vi "Builder.vi"() -> ()   [LabVIEW 2023]
uses:
  <vilib>/addons/_JKI Toolkits/State Machine/_JKI_lib_State_Machine.llb/Select State(s)_err__jki_lib_state_machine.vi
  <vilib>/AppBuilder/AB_API_Simple/Build (path).vi
  <userlib>/_OpenG.lib/appcontrol/appcontrol.llb/openg_application_control.lvlib
  <vilib>/AppBuilder/AB_API_Simple/NI_App_Builder_API.lvlib
panel:
  in  "BUILDER STATUS":i32(listbox)
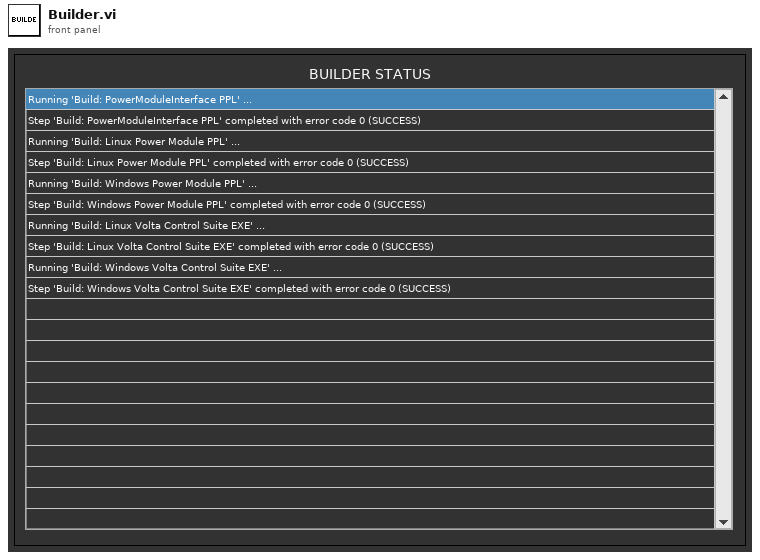
[diagram p1: front panel]
types:
  T1 = enum32{"Invalid", "Standard", "Closed", "Hidden", "Minimized", "Maximized"}
  T2 = enum32{"invalid app kind", "Development System", "Run Time System", "Student Edition", "Embedded LabVIEW", "Evaluation", "Custom"}
  T3 = cluster{"Core":cluster{"Current VI Reference":refnum<vi>, "Close Panel on Exit?":bool}}
  T4 = cluster{"Current VI Reference":refnum<vi>, "Close Panel on Exit?":bool}
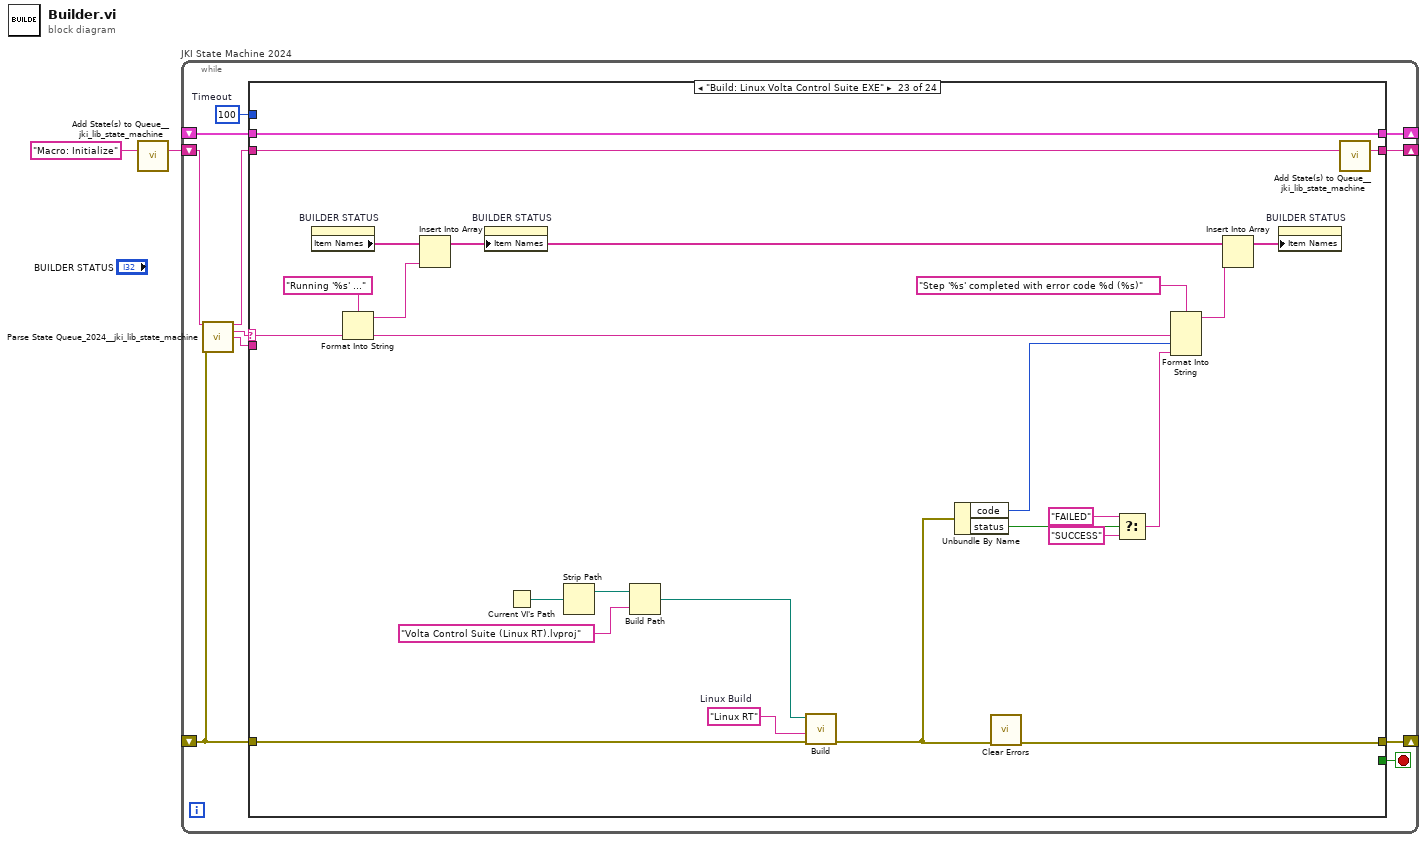
[diagram p0: block diagram]
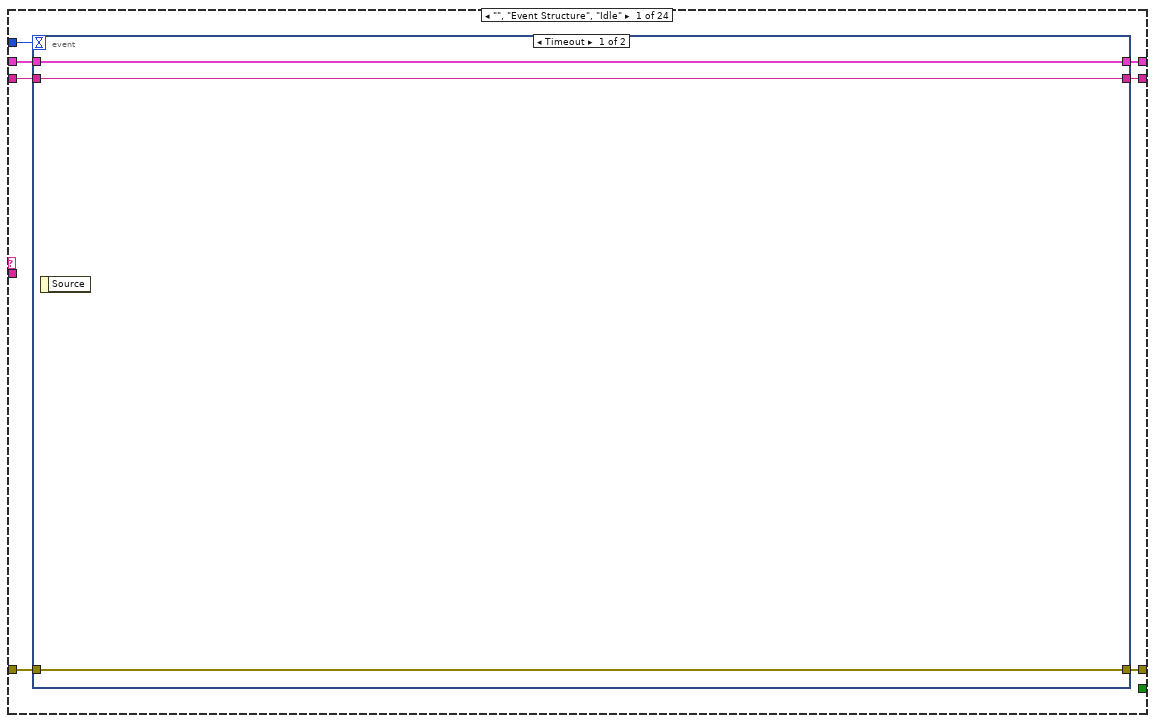
[diagram p2: hidden frame]
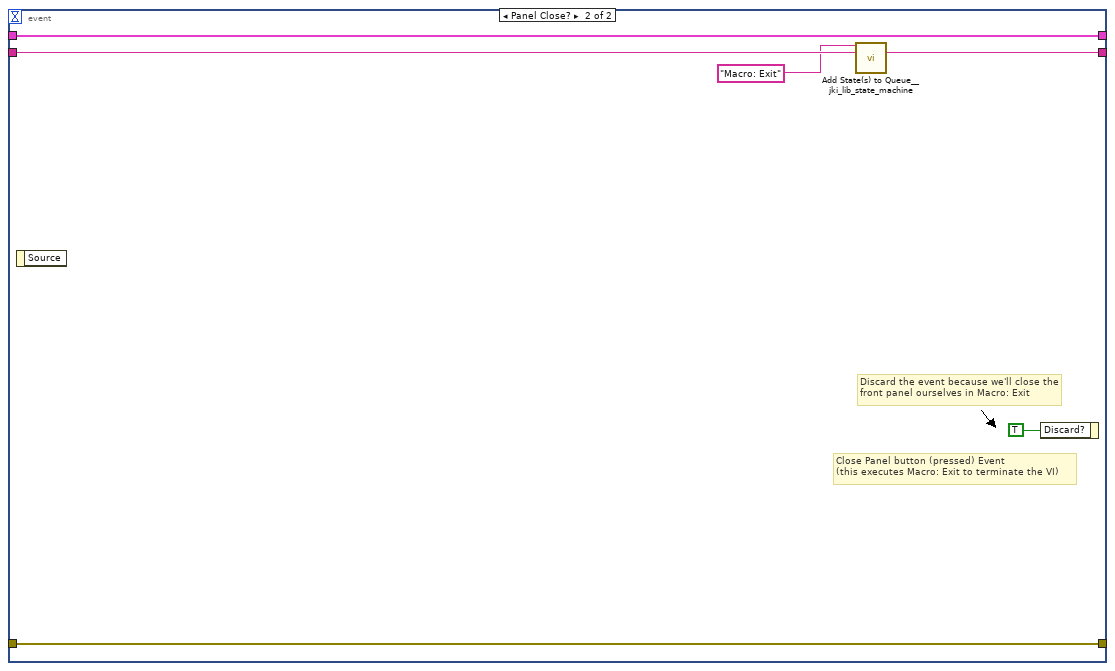
[diagram p3: hidden frame]
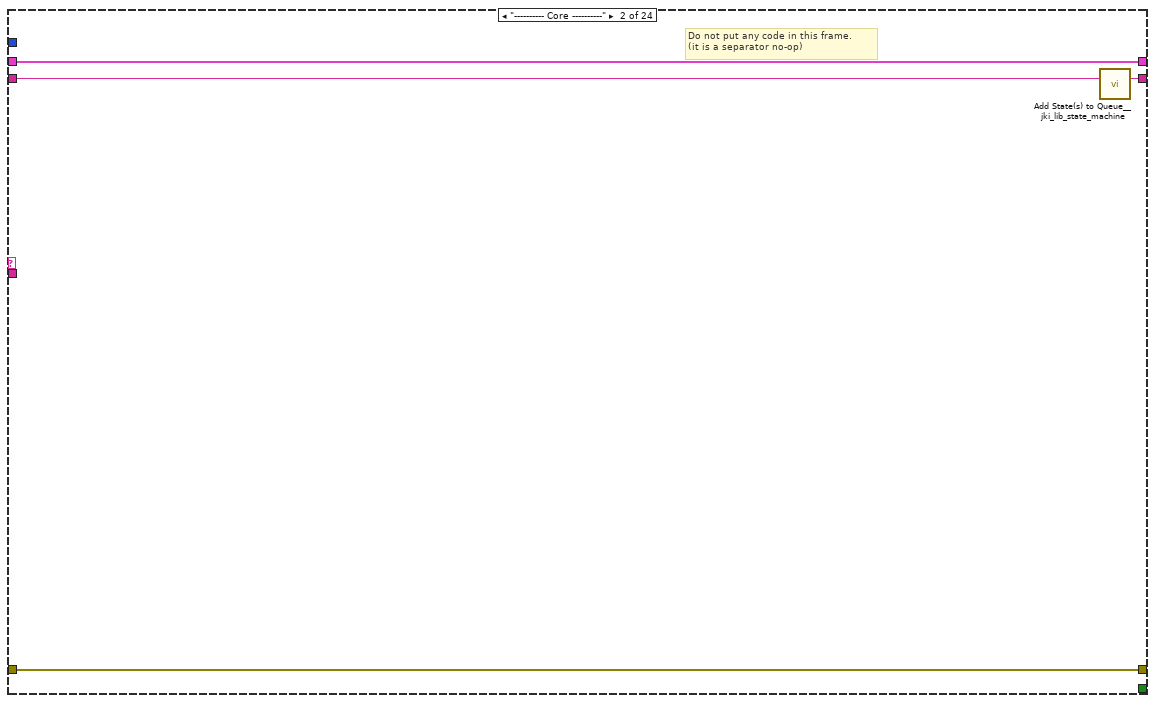
[diagram p4: hidden frame]
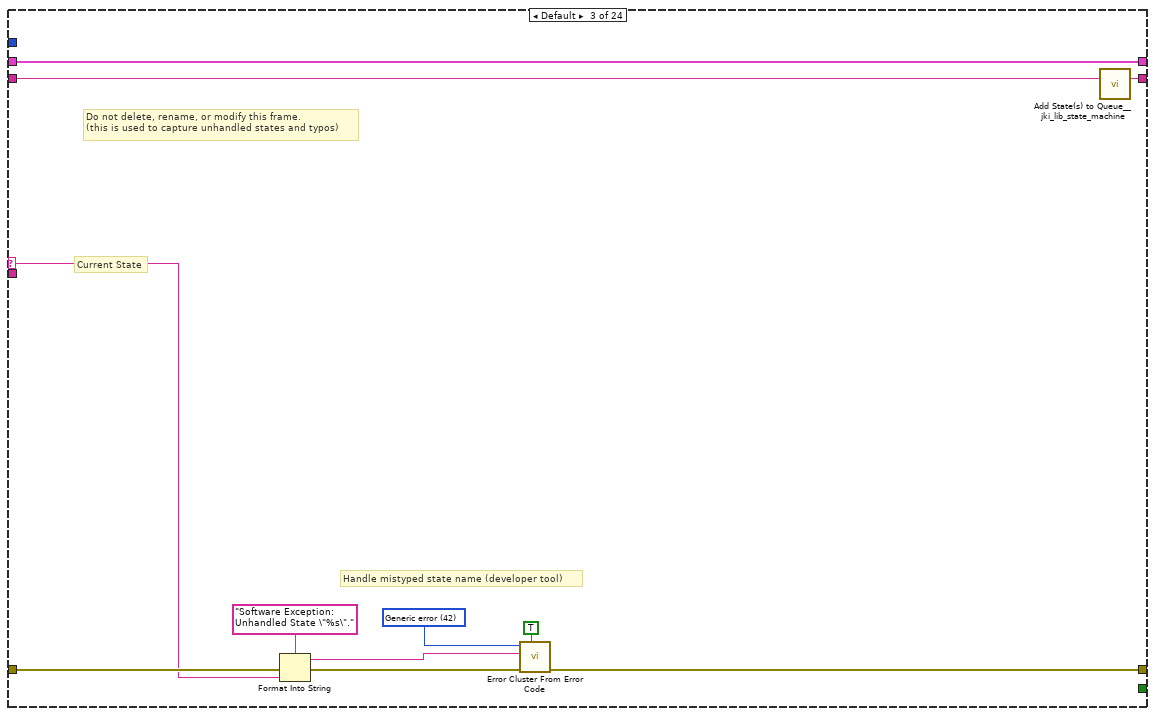
[diagram p5: hidden frame]
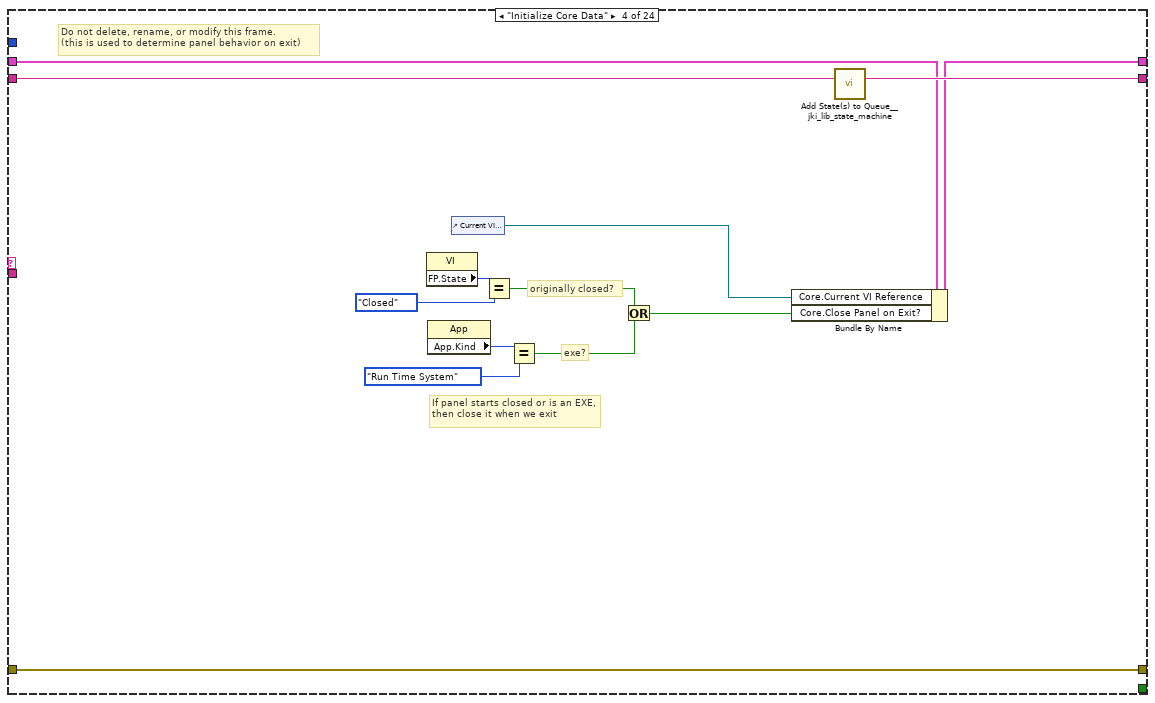
[diagram p6: hidden frame]
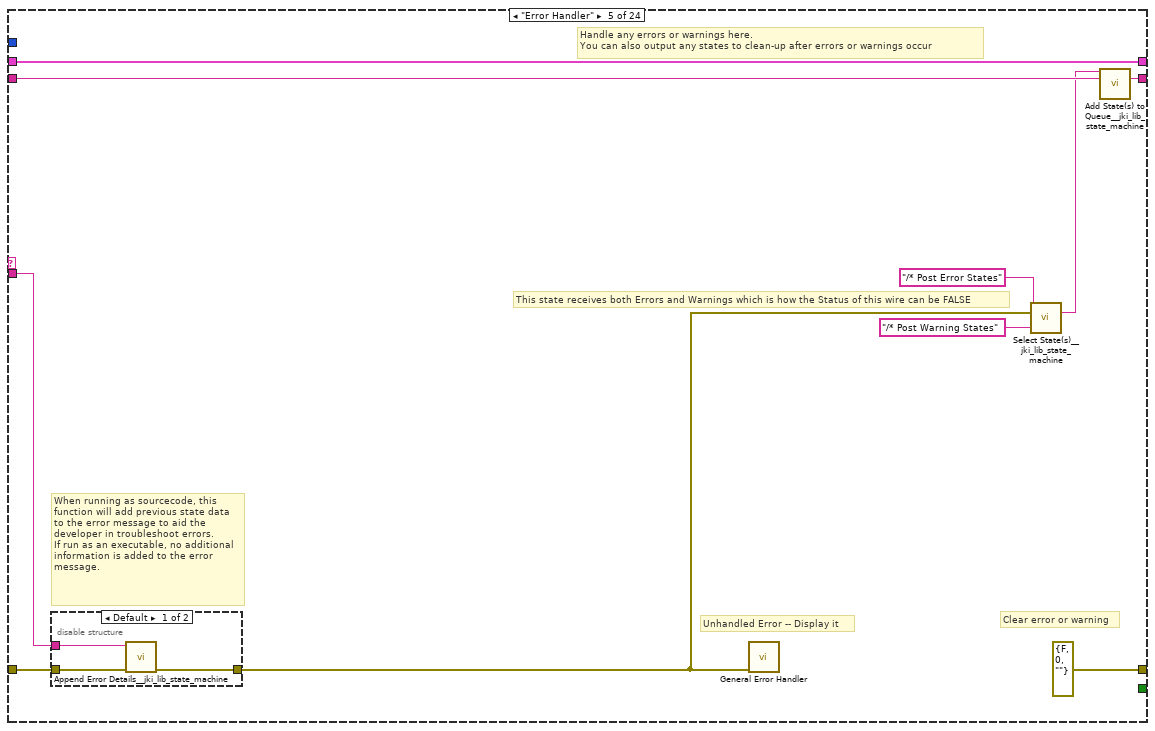
[diagram p7: hidden frame]
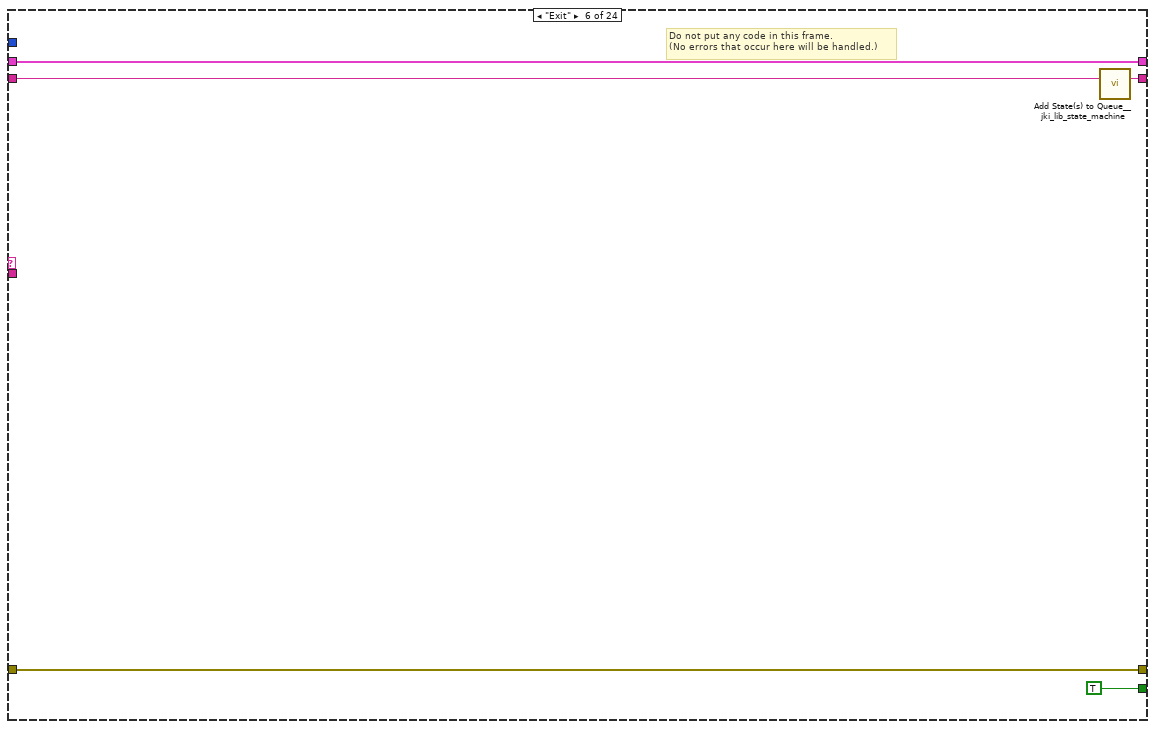
[diagram p9: hidden frame]
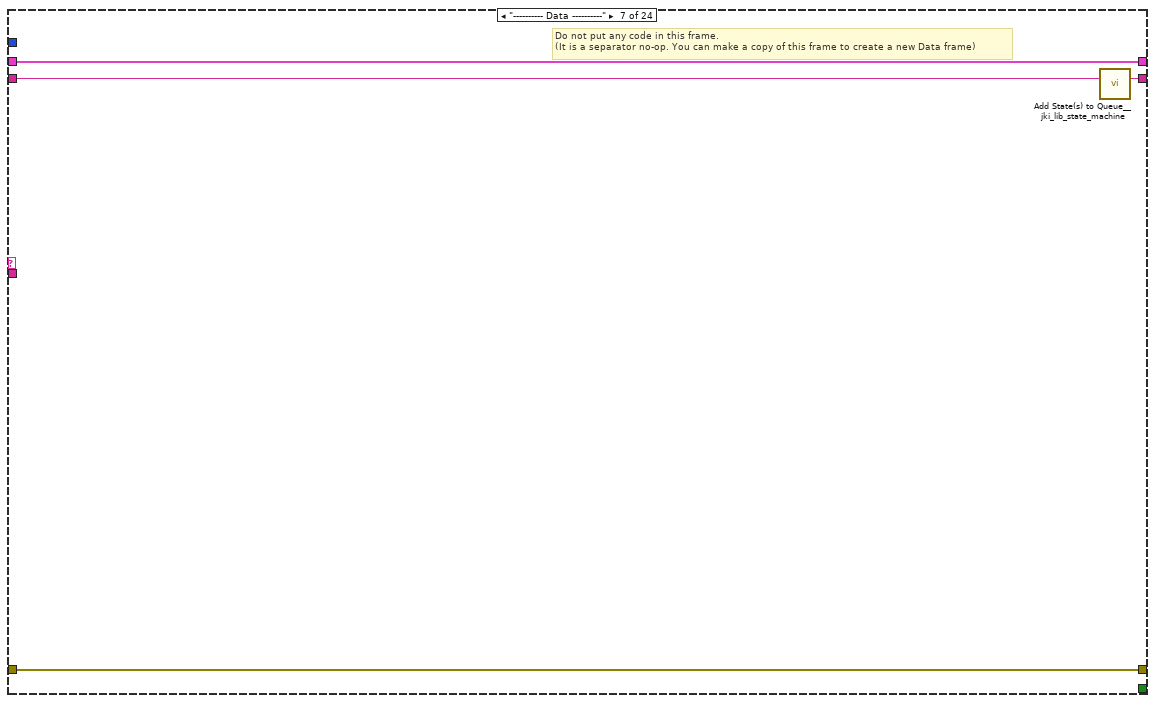
[diagram p10: hidden frame]
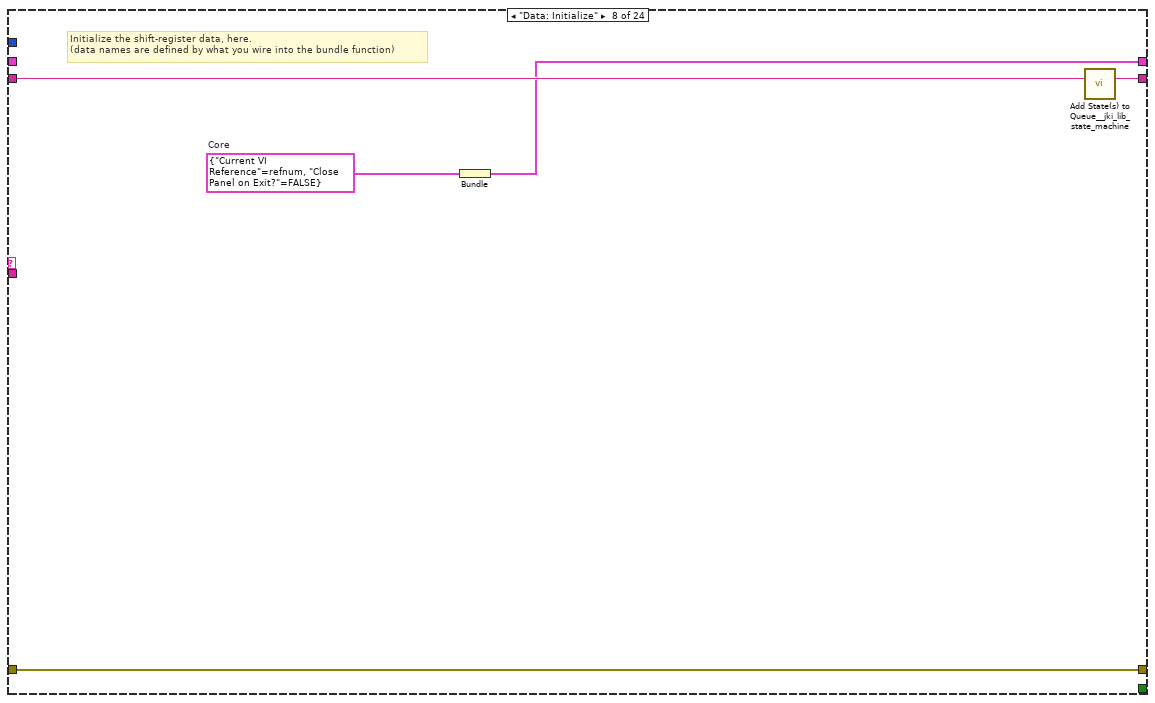
[diagram p11: hidden frame]
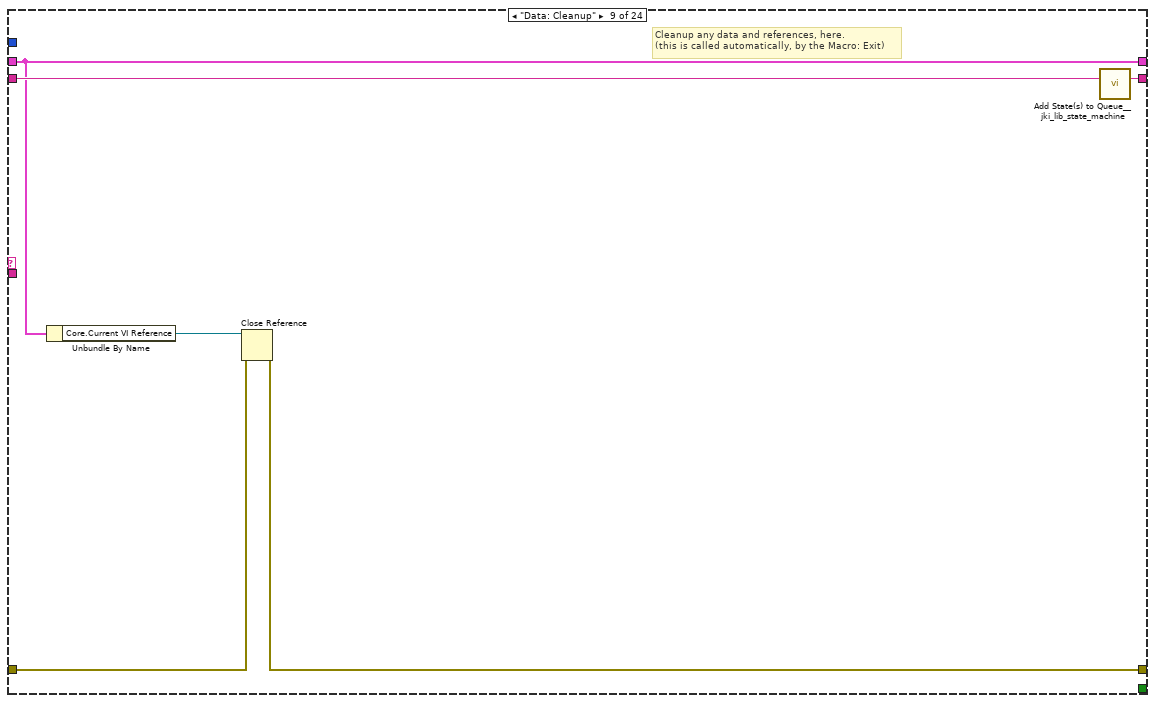
[diagram p12: hidden frame]
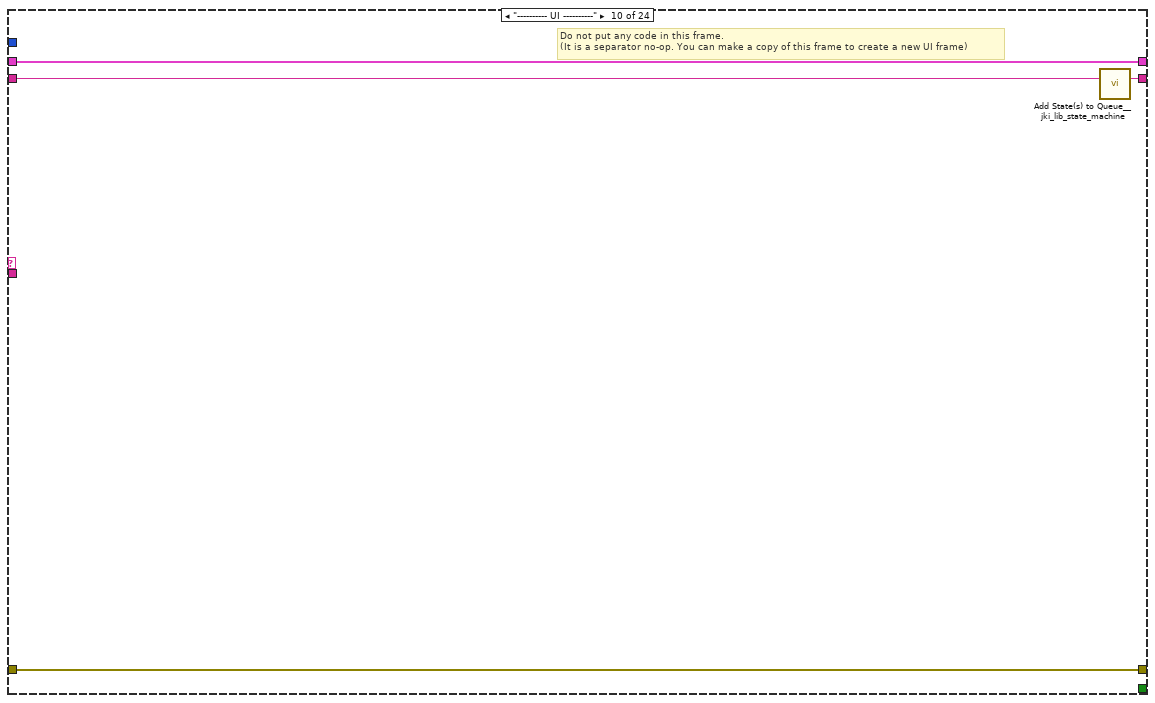
[diagram p13: hidden frame]
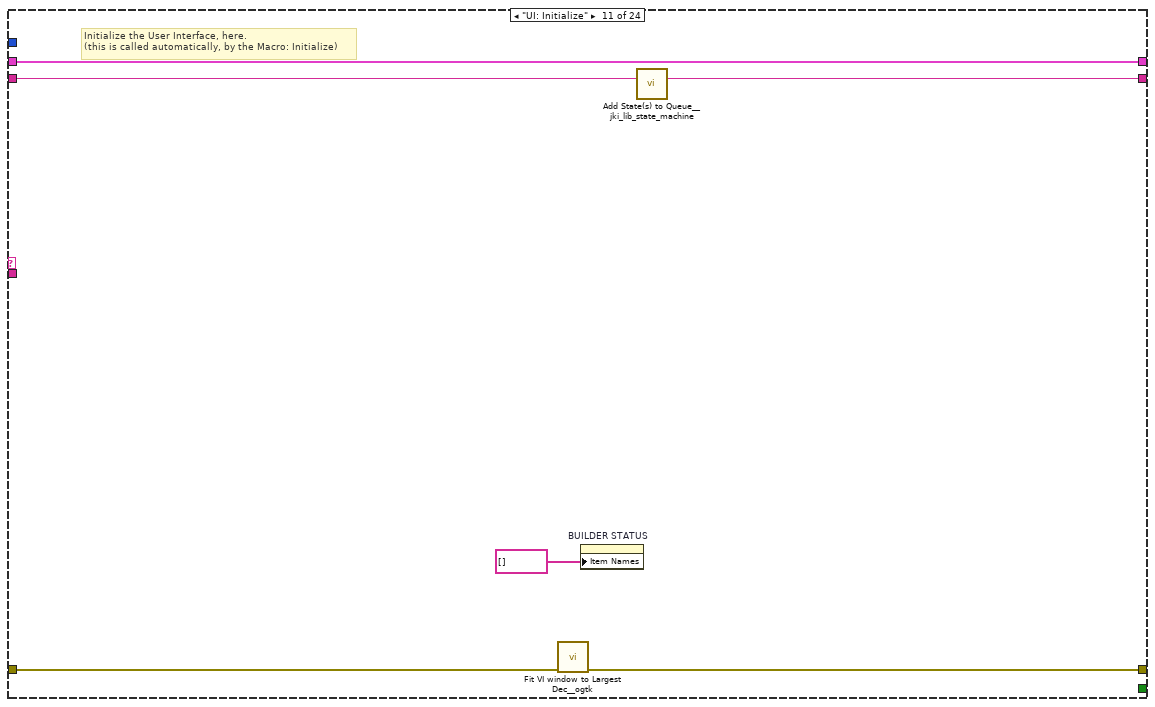
[diagram p14: hidden frame]
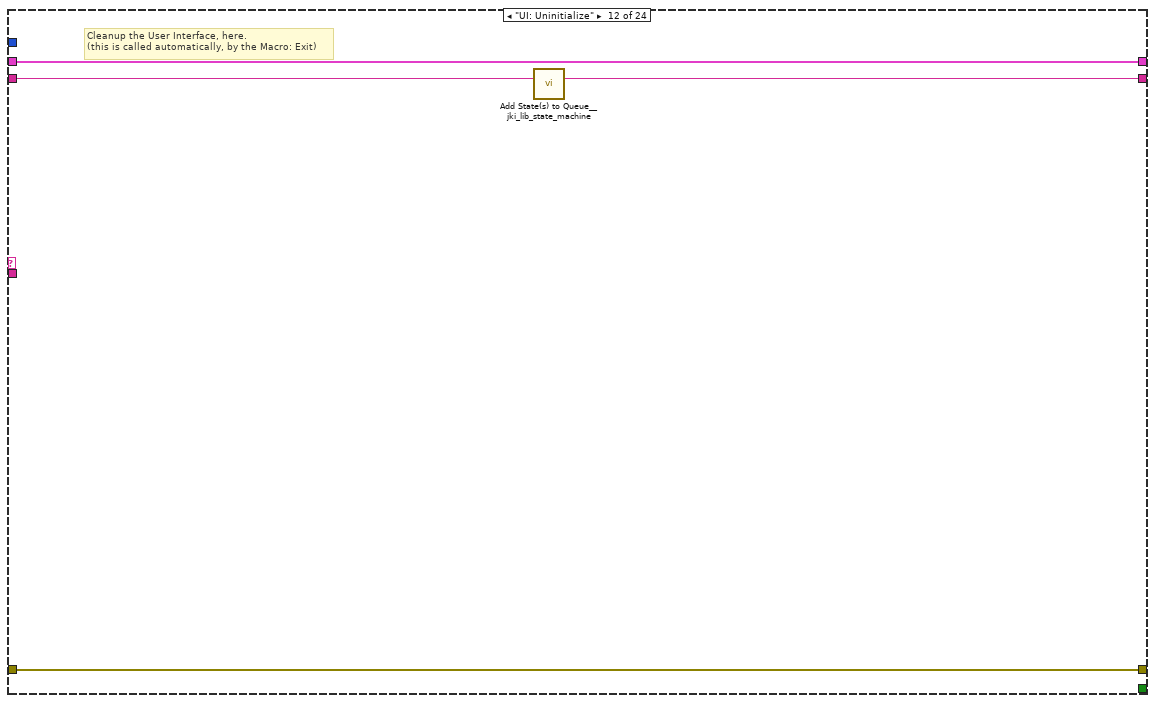
[diagram p15: hidden frame]
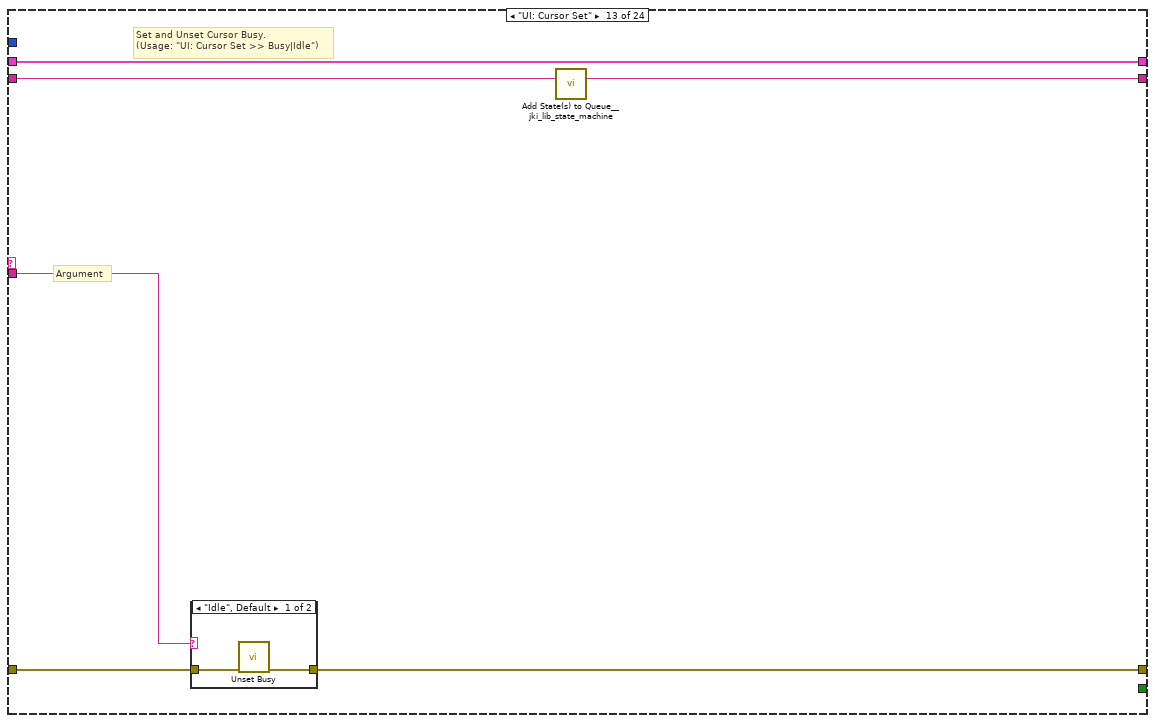
[diagram p16: hidden frame]
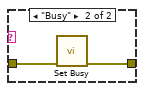
[diagram p17: hidden frame]
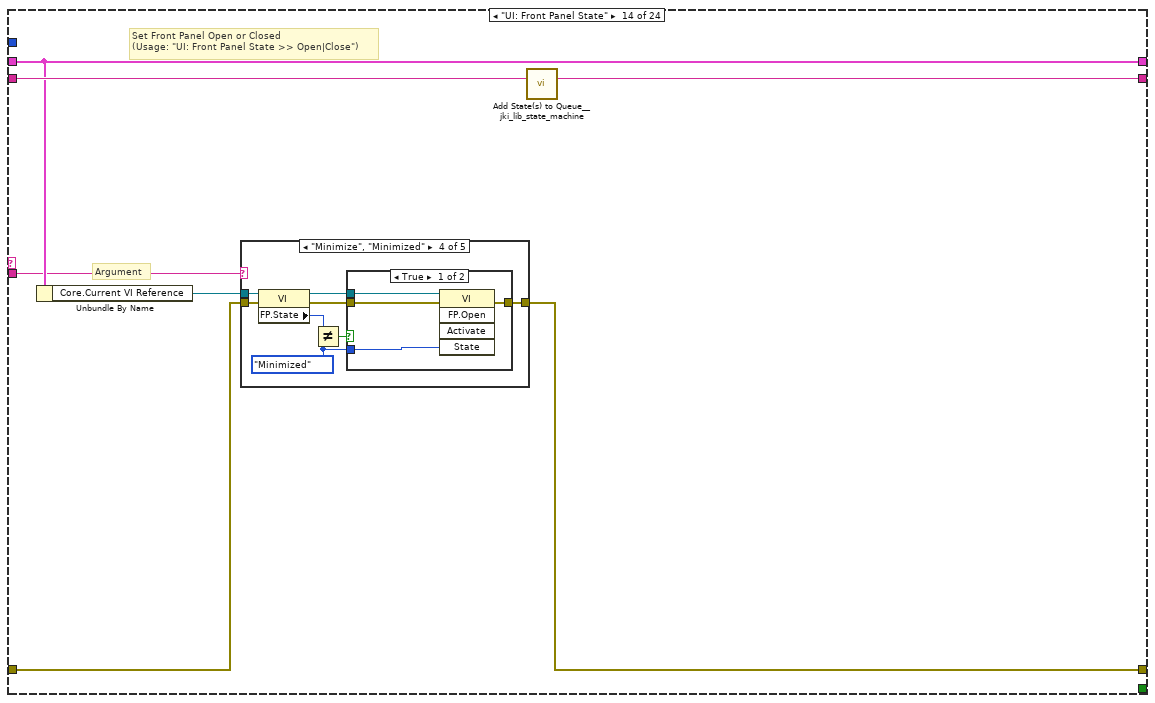
[diagram p18: hidden frame]
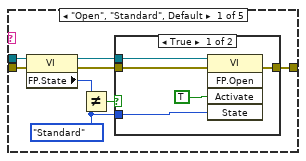
[diagram p19: hidden frame]
diagram:
  n1 = call <vilib>:"Add State(s) to Queue__jki_lib_state_machine.vi"("State(s) in (\"\")"="Macro: Initialize") -> ("States Out"=w2:string)  [unwired: 14 in]
  n2 = while "JKI State Machine 2024" {
    shift-right: [w6] -> _
    shift-left: _ -> [w5]
    shift-right: [w9] -> _
    shift-left: _ -> [w3]
    shift-right: [w8] -> _
    shift-left: w2 -> [w10]
    stop <- w7 stop-if-true
    w4 = 100  # Timeout
    n3 = call <vilib>:"Parse State Queue_2024__jki_lib_state_machine.vi"("State Queue"=w10, "Error In (no error)"=w3) -> ("Remaining States"=w12:string, "Current State"=w13:string, "Arguments"=w11:string)  [unwired: 11 in]
    n4 = case shown="\"Build: Linux Volta Control Suite EXE\"" w13 {
      selector: w13 -> [_ _ w34 _ _ _ _ _ _ _ _ _ _ _ _ _ _ _ _ w230 w253 w277 w301 w325]
      tunnel: w12 -> [w20 w33 w38 w57 w67 w76 w80 w85 w91 w95 w101 w105 w111 w122 w191 w196 w201 w206 w210 w238 w262 w286 w310 w334]
      tunnel: w11 -> [_ _ _ _ w62 _ _ _ _ _ _ _ w106 w116 _ _ _ _ _ _ _ _ _ _]
      tunnel: w5 -> [w18 w30 w36 w50 w64 w74 w77 _ w86 w92 w99 w103 w109 w118 w188 w193 w198 w204 w207 w236 w260 w284 w308 w332]
      tunnel: [w17 w31 w40 w54 errorcluster {"status"=FALSE, "code"=0, "source"=""} ("error out") w73 w78 w82 w87 w93 w96 w102 w107 w119 w189 w194 w199 w203 w208 w218 w246 w270 w294 w318] -> w9
      tunnel: w3 -> [w14 w31 w39 w54 w63 w73 w78 w82 w88 w93 w98 w102 w108 w120 w189 w194 w199 w203 w208 w225 w244 w268 w292 w316]
      tunnel: [w19 w32 w37 w56 w66 w75 w79 w84 w90 w94 w100 w104 w110 w121 w190 w195 w200 w205 w209 w237 w261 w285 w309 w333] -> w8
      tunnel: [_ _ _ _ _ TRUE _ _ _ _ _ _ _ _ _ _ _ _ _ _ _ _ _ _] -> w7
      tunnel: [w16 w30 w36 w55 w64 w74 w77 w83 w86 w92 w99 w103 w109 w118 w188 w193 w198 w204 w207 w236 w260 w284 w308 w332] -> w6
      tunnel: w4 -> [w15 _ _ _ _ _ _ _ _ _ _ _ _ _ _ _ _ _ _ _ _ _ _ _]
      frame "", "Event Structure", "Idle" {
        n5 = event shown="[0] Timeout" {
          selector: _ -> [_ _]
          dyn-events: _ -> [_ _]
          timeout: w15 -> [_ _]
          tunnel: w20 -> [w21 w29]
          tunnel: [w21 w28] -> w19
          tunnel: w18 -> [w22 w26]
          tunnel: [w23 w27] -> w17
          tunnel: w14 -> [w23 w27]
          tunnel: [w22 w26] -> w16
          event Timeout {
            n6 = event-data() -> ()  [unwired: 1 in, 1 out]
          }
          event Panel Close? {
            # "Discard the event because we'll close the front panel ourselves in Macro: Exit"
            # "Close Panel button (pressed) Event\n(this executes Macro: Exit to terminate the VI)"
            n7 = event-data() -> ()  [unwired: 1 in, 1 out]
            n8 = call <vilib>:"Add State(s) to Queue__jki_lib_state_machine.vi"("State(s) in Front (\"\")"="Macro: Exit", "State(s) in (\"\")"=w29) -> ("States Out"=w28:string)  [unwired: 13 in]
            n9 = event-data("Discard?"=TRUE) -> ()  [unwired: 1 in, 1 out]
          }
        }
      }
      frame "---------- Core ----------" {
        # "Do not put any code in this frame.\n(it is a separator no-op)"
        n10 = call <vilib>:"Add State(s) to Queue__jki_lib_state_machine.vi"("State(s) in (\"\")"=w33) -> ("States Out"=w32:string)  [unwired: 14 in]
      }
      frame Default {
        w43 = 42 items=["No error", "Argument error", "Memory is full", "Out of zone", "End of file", "File already open", "Generic file I/O error", "File not found", "File permission error", "Disk is full", "Duplicate path", "Too many files open", "System feature not enabled", "Resource file not found", "Cannot add resource", "Resource not found", "Image not found", "Image memory error", "Pen does not exist", "Config type invalid", "Config token not found", "Config parse error", "Config memory error", "Bad external code format", "Bad external code offset", "External code not present", "Null window", "Destroy window error", "Null menu", "Print aborted", "Bad print record", "Print driver error", "Windows error during printing", "Memory error during printing", "Print dialog error", "Generic print error", "Invalid device refnum", "Device not found", "Device parameter error", "Device unit error", "Cannot open device", "Device call aborted", "Generic error", "Cancelled by user", "Object ID too low", "Object ID too high", "Object not in heap", "Unknown heap", "Unknown object (invalid DefProc)", "Unknown object (DefProc not in table)", "Message out of range", "Invalid (null) method", "Unknown message", "Manager call not supported", "Bad address", "Network operation in progress", "Network operation timed out", "Connection is busy", "Network attribute not supported", "Network error", "Address in use", "System out of memory", "Connection aborted", "Connection refused", "Not connected", "Already connected", "Connection closed", "Initialization error (interapplication manager)", "Bad occurrence", "Wait on unbound occurrence handler", "Occurrence queue overflow", "Datalog type conflict", "Unused", "Unrecognized type (interapplication manager)", "Memory corrupt", "Failed to make temporary DLL", "Old CIN version", "Drag socket not found", "Failed to load drop-object", "Failed to register OLE object", "Failed to release OLE object", "Format specifier type mismatch", "Unknown format specifier", "Too few format specifiers", "Too many format specifiers", "Scan failed", "Newer CIN version", "Error converting to variant", "Runtime menu error", "Password tampered", "Variant attribute not found", "Incompatible variant data type", "Event data is not available", "Event Store is not present", "Occurrence is not found", "Event Queue is not created", "Event info is not available", "Refnum passed is NULL", "Error retrieving Class GUID", "Error retrieving CoClass GUID", "Error retrieving TypeLib GUID.", "Bad built application magic bytes.", "Specific driver is different from the specific driver associated with the Logical Name.", "There is no session opened to the class driver.", "Max Error", "MAX - Error with config objects", "MAX - Error loading configuration", "MAX - Group not supported"]
        # "Current State"
        # "Do not delete, rename, or modify this frame.\n(this is used to capture unhandled states and typos)"
        # "Handle mistyped state name (developer tool)"
        n11 = Format Into String(format string="Software Exception: Unhandled State \"%s\"." ("message"), error in=w39, w34) -> (resulting string=w42:string, error out=w41:errorcluster)  [unwired: 1 in]
        n12 = call <vilib>:"Error Cluster From Error Code.vi"("show call chain? (False)"=TRUE, "error in (no error)"=w41, "error message (\"\")"=w42, "error code (0)"=w43) -> ("error out"=w40:errorcluster)  [unwired: 5 in]
        n13 = call <vilib>:"Add State(s) to Queue__jki_lib_state_machine.vi"("State(s) in (\"\")"=w38) -> ("States Out"=w37:string)  [unwired: 14 in]
      }
      frame "Initialize Core Data" {
        # "Do not delete, rename, or modify this frame.\n(this is used to determine panel behavior on exit)"
        # "originally closed?"
        # "exe?"
        # "If panel starts closed or is an EXE, then close it when we exit"
        n14 = property class="VI"() -> ("FP.State"=w47:T1)  [unwired: 2 in, 2 out]
        n15 = property class="App"() -> ("App.Kind"=w53:T2)  [unwired: 2 in, 2 out]
        n16 = control-ref of="Current VI Reference"() -> (w48:refnum<vi>)
        n17 = Equal?(x=w47, y=T1."Closed" ("Front Panel Window:State")) -> (x = y?=w45:bool)
        n18 = Equal?(x=w53, y=T2."Run Time System" ("Application:Kind")) -> (x = y?=w51:bool)
        n19 = Or(x=w45, y=w51) -> (x .or. y?=w49:bool)
        n20 = Bundle By Name(cluster=w50, "Core.Current VI Reference"=w48, "Core.Close Panel on Exit?"=w49) -> (w55:T3)
        n21 = call <vilib>:"Add State(s) to Queue__jki_lib_state_machine.vi"("State(s) in (\"\")"=w57) -> ("States Out"=w56:string)  [unwired: 14 in]
      }
      frame "Error Handler" {
        # "When running as sourcecode, this function will add previous state data to the error message to aid the developer in troubleshoot errors.\nIf run as an executable, no additional information is added to the error message."
        # "This state receives both Errors and Warnings which is how the Status of this wire can be FALSE"
        # "Unhandled Error -- Display it"
        # "Handle any errors or warnings here.\nYou can also output any states to clean-up after errors or warnings occur"
        # "Clear error or warning"
        n22 = disable-structure shown="Default" {
          disable-tunnel: w63 -> [w70 w71]
          disable-tunnel: w62 -> [w69 _]
          disable-tunnel: [w68 w71] -> w61
          frame condition #0 (active) {
            n23 = call <vilib>:"Append Error Details__jki_lib_state_machine.vi"("error in (no error)"=w70, "Previous State and Argument(s)"=w69) -> ("error out"=w68:errorcluster)  [unwired: 9 in]
          }
          frame condition #1 {
          }
        }
        n24 = call <vilib>:"General Error Handler.vi"("error in (no error)"=w61) -> ()  [unwired: 10 in, 5 out]
        n25 = call-poly <vilib>:"Select State(s)__jki_lib_state_machine.vi"("State(s) if True (\"\")"="/* Post Error States", "Select"=w61, "State(s) if False (\"\")"="/* Post Warning States") -> ("States Out"=w59:string)  [unwired: 12 in]
        n26 = call <vilib>:"Add State(s) to Queue__jki_lib_state_machine.vi"("State(s) in Front (\"\")"=w59, "State(s) in (\"\")"=w67) -> ("States Out"=w66:string)  [unwired: 13 in]
      }
      frame "Exit" {
        # "Do not put any code in this frame.\n(No errors that occur here will be handled.)"
        n27 = call <vilib>:"Add State(s) to Queue__jki_lib_state_machine.vi"("State(s) in (\"\")"=w76) -> ("States Out"=w75:string)  [unwired: 14 in]
      }
      frame "---------- Data ----------" {
        # "Do not put any code in this frame.\n(It is a separator no-op. You can make a copy of this frame to create a new Data frame)"
        n28 = call <vilib>:"Add State(s) to Queue__jki_lib_state_machine.vi"("State(s) in (\"\")"=w80) -> ("States Out"=w79:string)  [unwired: 14 in]
      }
      frame "Data: Initialize" {
        w81 = T4 {"Current VI Reference"=refnum, "Close Panel on Exit?"=FALSE}  # Core
        # "Initialize the shift-register data, here.\n(data names are defined by what you wire into the bundle function)"
        n29 = Bundle("Core"=w81) -> (w83:T3)  [unwired: 1 in]
        n30 = call <vilib>:"Add State(s) to Queue__jki_lib_state_machine.vi"("State(s) in (\"\")"=w85) -> ("States Out"=w84:string)  [unwired: 14 in]
      }
      frame "Data: Cleanup" {
        # "Cleanup any data and references, here.\n(this is called automatically, by the Macro: Exit)"
        n31 = Unbundle By Name(w86) -> ("Core.Current VI Reference"=w89:refnum<vi>)
        n32 = Close Reference(reference=w89, error in (no error)=w88) -> (error out=w87:errorcluster)
        n33 = call <vilib>:"Add State(s) to Queue__jki_lib_state_machine.vi"("State(s) in (\"\")"=w91) -> ("States Out"=w90:string)  [unwired: 14 in]
      }
      frame "---------- UI ----------" {
        # "Do not put any code in this frame.\n(It is a separator no-op. You can make a copy of this frame to create a new UI frame)"
        n34 = call <vilib>:"Add State(s) to Queue__jki_lib_state_machine.vi"("State(s) in (\"\")"=w95) -> ("States Out"=w94:string)  [unwired: 14 in]
      }
      frame "UI: Initialize" {
        # "Initialize the User Interface, here.\n(this is called automatically, by the Macro: Initialize)"
        n35 = call <userlib>:"Fit VI window to Largest Dec__ogtk.vi"("error in (no error)"=w98) -> ("error out"=w96:errorcluster)  [unwired: 5 in, 1 out]
        n36 = property on="BUILDER STATUS" class="LstBox (strict)"("Item Names"=string[] []) -> ()  [unwired: 2 in, 2 out]
        n37 = call <vilib>:"Add State(s) to Queue__jki_lib_state_machine.vi"("State(s) in (\"\")"=w101) -> ("States Out"=w100:string)  [unwired: 14 in]
      }
      frame "UI: Uninitialize" {
        # "Cleanup the User Interface, here.\n(this is called automatically, by the Macro: Exit)"
        n38 = call <vilib>:"Add State(s) to Queue__jki_lib_state_machine.vi"("State(s) in (\"\")"=w105) -> ("States Out"=w104:string)  [unwired: 14 in]
      }
      frame "UI: Cursor Set" {
        # "Argument"
        # "Set and Unset Cursor Busy.\n(Usage: \"UI: Cursor Set >> Busy|Idle\")"
        n39 = case shown="\"Idle\", Default" w106 {
          tunnel: w108 -> [w113 w115]
          tunnel: [w112 w114] -> w107
          frame "Idle", Default {
            n40 = call <vilib>:"Unset Busy.vi"("error in (no error)"=w113) -> ("error out"=w112:errorcluster)  [unwired: 10 in]
          }
          frame "Busy" {
            n41 = call <vilib>:"Set Busy.vi"("error in (no error)"=w115) -> ("error out"=w114:errorcluster)  [unwired: 9 in, 1 out]
          }
        }
        n42 = call <vilib>:"Add State(s) to Queue__jki_lib_state_machine.vi"("State(s) in (\"\")"=w111) -> ("States Out"=w110:string)  [unwired: 14 in]
      }
      frame "UI: Front Panel State" {
        # "Argument"
        # "Set Front Panel Open or Closed\n(Usage: \"UI: Front Panel State >> Open|Close\")"
        n43 = Unbundle By Name(w118) -> ("Core.Current VI Reference"=w117:refnum<vi>)
        n44 = case shown="\"Minimize\", \"Minimized\"" w116 {
          tunnel: w120 -> [w128 w143 w154 w167 w180]
          tunnel: [w130 w144 w156 w169 w182] -> w119
          tunnel: w117 -> [w129 w141 w155 w168 w181]
          frame "Open", "Standard", Default {
            w123 = T1."Standard" ("State")
            n45 = property class="VI"(reference=w129, error in=w128) -> (reference out=w126:refnum<vi>, error out=w127:errorcluster, "FP.State"=w125:T1)
            n46 = Not Equal?(x=w125, y=w123) -> (x != y?=w124:bool)
            n47 = case shown="True" w124 {
              tunnel: [w134 w136] -> w130
              tunnel: w127 -> [w133 w136]
              tunnel: w126 -> [w132 _]
              tunnel: w123 -> [w131 _]
              frame True {
                n48 = invoke class="VI" method="FP.Open"(reference=w132, error in=w133, "Activate"=TRUE, "State"=w131) -> (error out=w134:errorcluster)  [unwired: 1 in, 4 out]
              }
              frame False {
              }
            }
          }
          frame "Close", "Closed" {
            n49 = property class="VI"(reference=w141, error in=w143) -> (reference out=w140:refnum<vi>, error out=w142:errorcluster, "FP.State"=w138:T1)
            n50 = Not Equal?(x=w138, y=T1."Closed" ("Front Panel Window:State")) -> (x != y?=w137:bool)
            n51 = case shown="True" w137 {
              tunnel: [w145 w148] -> w144
              tunnel: w142 -> [w145 w147]
              tunnel: w140 -> [_ w146]
              frame False {
              }
              frame True {
                n52 = invoke class="VI" method="FP.Close"(reference=w146, error in=w147) -> (error out=w148:errorcluster)  [unwired: 1 in, 2 out]
              }
            }
          }
          frame "Hidden", "Hide" {
            w149 = T1."Hidden" ("State")
            n53 = property class="VI"(reference=w155, error in=w154) -> (reference out=w152:refnum<vi>, error out=w153:errorcluster, "FP.State"=w151:T1)
            n54 = Not Equal?(x=w151, y=w149) -> (x != y?=w150:bool)
            n55 = case shown="True" w150 {
              tunnel: [w160 w161] -> w156
              tunnel: w153 -> [w159 w161]
              tunnel: w152 -> [w158 _]
              tunnel: w149 -> [w157 _]
              frame True {
                n56 = invoke class="VI" method="FP.Open"(reference=w158, error in=w159, "State"=w157) -> (error out=w160:errorcluster)  [unwired: 2 in, 4 out]
              }
              frame False {
              }
            }
          }
          frame "Minimize", "Minimized" {
            w162 = T1."Minimized" ("State")
            n57 = property class="VI"(reference=w168, error in=w167) -> (reference out=w165:refnum<vi>, error out=w166:errorcluster, "FP.State"=w164:T1)
            n58 = Not Equal?(x=w164, y=w162) -> (x != y?=w163:bool)
            n59 = case shown="True" w163 {
              tunnel: [w173 w174] -> w169
              tunnel: w166 -> [w172 w174]
              tunnel: w165 -> [w171 _]
              tunnel: w162 -> [w170 _]
              frame True {
                n60 = invoke class="VI" method="FP.Open"(reference=w171, error in=w172, "State"=w170) -> (error out=w173:errorcluster)  [unwired: 2 in, 4 out]
              }
              frame False {
              }
            }
          }
          frame "Maximize", "Maximized" {
            w175 = T1."Maximized" ("State")
            n61 = property class="VI"(reference=w181, error in=w180) -> (reference out=w178:refnum<vi>, error out=w179:errorcluster, "FP.State"=w177:T1)
            n62 = Not Equal?(x=w177, y=w175) -> (x != y?=w176:bool)
            n63 = case shown="True" w176 {
              tunnel: [w186 w187] -> w182
              tunnel: w179 -> [w185 w187]
              tunnel: w178 -> [w184 _]
              tunnel: w175 -> [w183 _]
              frame True {
                n64 = invoke class="VI" method="FP.Open"(reference=w184, error in=w185, "State"=w183) -> (error out=w186:errorcluster)  [unwired: 2 in, 4 out]
              }
              frame False {
              }
            }
          }
        }
        n65 = call <vilib>:"Add State(s) to Queue__jki_lib_state_machine.vi"("State(s) in (\"\")"=w122) -> ("States Out"=w121:string)  [unwired: 14 in]
      }
      frame "---------- Macro ----------" {
        # "Do not put any code in this frame.\n(It is a separator no-op. You can make a copy of this frame to create a new Macro frame)"
        n66 = call <vilib>:"Add State(s) to Queue__jki_lib_state_machine.vi"("State(s) in (\"\")"=w191) -> ("States Out"=w190:string)  [unwired: 14 in]
      }
      frame "Macro: Initialize" {
        w192 = "Data: Initialize\nInitialize Core Data\nUI: Initialize\nUI: Front Panel State >> Open\nMacro: Run"  # Data: Initialize Initialize Core Data UI: Initialize UI: Front Panel State >> Open Macro: Run
        # "Initialization Macro\n(This is called once, when the VI starts)"
        n67 = call <vilib>:"Add State(s) to Queue__jki_lib_state_machine.vi"("State(s) in Front (\"\")"=w192, "State(s) in (\"\")"=w196) -> ("States Out"=w195:string)  [unwired: 13 in]
      }
      frame "Macro: Run" {
        w197 = "Build: PowerModuleInterface PPL\nBuild: Linux Power Module PPL\nBuild: Windows Power Module PPL\nBuild: Linux Volta Control Suite EXE\nBuild: Windows Volta Control Suite EXE\nMacro: Exit"  # Build: PowerModuleInterface PPL Build: Linux Power Module PPL Build: Windows Power Module PPL Build: Linux Volta Control Suite EXE Build: Windows Volta Control Suite EXE Macro: Exit
        # "Run Macro\n(This is called once, when the VI starts)"
        n68 = call <vilib>:"Add State(s) to Queue__jki_lib_state_machine.vi"("State(s) in Front (\"\")"=w197, "State(s) in (\"\")"=w201) -> ("States Out"=w200:string)  [unwired: 13 in]
      }
      frame "Macro: Exit" {
        # "Exit Macro\n(This is called once, when the VI exits)"
        n69 = call <vilib>:"Add State(s) to Queue__jki_lib_state_machine.vi"("State(s) in Front (\"\")"="UI: Uninitialize\nData: Cleanup\nExit", "State(s) in (\"\")"=w206) -> ("States Out"=w205:string)  [unwired: 13 in]
      }
      frame "---------- BUILD ----------" {
        # "Template Separator\n(You can make a copy of, or modify, this frame)"
        n70 = call <vilib>:"Add State(s) to Queue__jki_lib_state_machine.vi"("State(s) in (\"\")"=w210) -> ("States Out"=w209:string)  [unwired: 14 in]
      }
      frame "Build: PowerModuleInterface PPL" {
        w223 = "Linux RT"  # Linux Build
        w224 = "My Computer"  # Windows Build
        n71 = property on="BUILDER STATUS" class="LstBox (strict)"() -> ("Item Names"=w235:string[])  [unwired: 2 in, 2 out]
        n72 = Format Into String(format string="Running '%s' ...", w230) -> (resulting string=w233:string)  [unwired: 2 in, 1 out]
        n73 = Current VI's Path() -> (path=w228:path)
        n74 = Insert Into Array(array=w235, new element=w233) -> (w232:string[])  [unwired: 1 in]
        n75 = Strip Path(path=w228) -> (stripped path=w227:path)  [unwired: 1 out]
        n76 = property on="BUILDER STATUS" class="LstBox (strict)"("Item Names"=w232) -> ()  [unwired: 2 in, 2 out]
        n77 = Build Path(base path=w227, name or relative path="PowerModuleInterface.lvproj") -> (appended path=w222:path)
        n78 = call-poly <vilib>:"Build.vi"("error in (no error)"=w225, "Name of target (My Computer)"=w224, "Path to project"=w222) -> ("error out"=w220:errorcluster)  [unwired: 7 in, 1 out]
        n79 = call <vilib>:"Clear Errors.vi"("error in (no error)"=w220) -> ("error out"=w221:errorcluster)  [unwired: 5 in, 1 out]
        n80 = call-poly <vilib>:"Build.vi"("error in (no error)"=w221, "Name of target (My Computer)"=w223, "Path to project"=w222) -> ("error out"=w219:errorcluster)  [unwired: 7 in, 1 out]
        n81 = Merge Errors(w220, w219) -> (w217:errorcluster)
        n82 = call <vilib>:"Clear Errors.vi"("error in (no error)"=w219) -> ("error out"=w218:errorcluster)  [unwired: 5 in, 1 out]
        n83 = Unbundle By Name(w217) -> ("code"=w216:i32, "status"=w212:bool)
        n84 = Select(t="FAILED", s=w212, f="SUCCESS") -> (s? t:f=w211:string)
        n85 = Format Into String(format string="Step '%s' completed with error code %d (%s)", w230, w216, w211) -> (resulting string=w229:string)  [unwired: 2 in, 1 out]
        n86 = Insert Into Array(array=w232, new element=w229) -> (w231:string[])  [unwired: 1 in]
        n87 = property on="BUILDER STATUS" class="LstBox (strict)"("Item Names"=w231) -> ()  [unwired: 2 in, 2 out]
        n88 = call <vilib>:"Add State(s) to Queue__jki_lib_state_machine.vi"("State(s) in (\"\")"=w238) -> ("States Out"=w237:string)  [unwired: 14 in]
      }
      frame "Build: Linux Power Module PPL" {
        w248 = "Linux RT"  # Linux Build
        n89 = property on="BUILDER STATUS" class="LstBox (strict)"() -> ("Item Names"=w259:string[])  [unwired: 2 in, 2 out]
        n90 = Format Into String(format string="Running '%s' ...", w253) -> (resulting string=w257:string)  [unwired: 2 in, 1 out]
        n91 = Insert Into Array(array=w259, new element=w257) -> (w256:string[])  [unwired: 1 in]
        n92 = property on="BUILDER STATUS" class="LstBox (strict)"("Item Names"=w256) -> ()  [unwired: 2 in, 2 out]
        n93 = Current VI's Path() -> (path=w251:path)
        n94 = Strip Path(path=w251) -> (stripped path=w250:path)  [unwired: 1 out]
        n95 = Build Path(base path=w250, name or relative path="Power Modules (Linux RT).lvproj") -> (appended path=w247:path)
        n96 = call-poly <vilib>:"Build.vi"("error in (no error)"=w244, "Name of target (My Computer)"=w248, "Path to project"=w247) -> ("error out"=w245:errorcluster)  [unwired: 7 in, 1 out]
        n97 = Unbundle By Name(w245) -> ("code"=w243:i32, "status"=w242:bool)
        n98 = call <vilib>:"Clear Errors.vi"("error in (no error)"=w245) -> ("error out"=w246:errorcluster)  [unwired: 5 in, 1 out]
        n99 = Select(t="FAILED", s=w242, f="SUCCESS") -> (s? t:f=w239:string)
        n100 = Format Into String(format string="Step '%s' completed with error code %d (%s)", w253, w243, w239) -> (resulting string=w252:string)  [unwired: 2 in, 1 out]
        n101 = Insert Into Array(array=w256, new element=w252) -> (w255:string[])  [unwired: 1 in]
        n102 = property on="BUILDER STATUS" class="LstBox (strict)"("Item Names"=w255) -> ()  [unwired: 2 in, 2 out]
        n103 = call <vilib>:"Add State(s) to Queue__jki_lib_state_machine.vi"("State(s) in (\"\")"=w262) -> ("States Out"=w261:string)  [unwired: 14 in]
      }
      frame "Build: Windows Power Module PPL" {
        w272 = "My Computer"  # Windows Build
        n104 = property on="BUILDER STATUS" class="LstBox (strict)"() -> ("Item Names"=w283:string[])  [unwired: 2 in, 2 out]
        n105 = Format Into String(format string="Running '%s' ...", w277) -> (resulting string=w281:string)  [unwired: 2 in, 1 out]
        n106 = Insert Into Array(array=w283, new element=w281) -> (w280:string[])  [unwired: 1 in]
        n107 = property on="BUILDER STATUS" class="LstBox (strict)"("Item Names"=w280) -> ()  [unwired: 2 in, 2 out]
        n108 = Current VI's Path() -> (path=w275:path)
        n109 = Strip Path(path=w275) -> (stripped path=w274:path)  [unwired: 1 out]
        n110 = Build Path(base path=w274, name or relative path="Power Modules (Windows).lvproj") -> (appended path=w271:path)
        n111 = call-poly <vilib>:"Build.vi"("error in (no error)"=w268, "Name of target (My Computer)"=w272, "Path to project"=w271) -> ("error out"=w269:errorcluster)  [unwired: 7 in, 1 out]
        n112 = Unbundle By Name(w269) -> ("code"=w267:i32, "status"=w266:bool)
        n113 = call <vilib>:"Clear Errors.vi"("error in (no error)"=w269) -> ("error out"=w270:errorcluster)  [unwired: 5 in, 1 out]
        n114 = Select(t="FAILED", s=w266, f="SUCCESS") -> (s? t:f=w263:string)
        n115 = Format Into String(format string="Step '%s' completed with error code %d (%s)", w277, w267, w263) -> (resulting string=w276:string)  [unwired: 2 in, 1 out]
        n116 = Insert Into Array(array=w280, new element=w276) -> (w279:string[])  [unwired: 1 in]
        n117 = property on="BUILDER STATUS" class="LstBox (strict)"("Item Names"=w279) -> ()  [unwired: 2 in, 2 out]
        n118 = call <vilib>:"Add State(s) to Queue__jki_lib_state_machine.vi"("State(s) in (\"\")"=w286) -> ("States Out"=w285:string)  [unwired: 14 in]
      }
      frame "Build: Linux Volta Control Suite EXE" {
        w296 = "Linux RT"  # Linux Build
        n119 = property on="BUILDER STATUS" class="LstBox (strict)"() -> ("Item Names"=w307:string[])  [unwired: 2 in, 2 out]
        n120 = Format Into String(format string="Running '%s' ...", w301) -> (resulting string=w305:string)  [unwired: 2 in, 1 out]
        n121 = Insert Into Array(array=w307, new element=w305) -> (w304:string[])  [unwired: 1 in]
        n122 = property on="BUILDER STATUS" class="LstBox (strict)"("Item Names"=w304) -> ()  [unwired: 2 in, 2 out]
        n123 = Current VI's Path() -> (path=w299:path)
        n124 = Strip Path(path=w299) -> (stripped path=w298:path)  [unwired: 1 out]
        n125 = Build Path(base path=w298, name or relative path="Volta Control Suite (Linux RT).lvproj") -> (appended path=w295:path)
        n126 = call-poly <vilib>:"Build.vi"("error in (no error)"=w292, "Name of target (My Computer)"=w296, "Path to project"=w295) -> ("error out"=w293:errorcluster)  [unwired: 7 in, 1 out]
        n127 = Unbundle By Name(w293) -> ("code"=w291:i32, "status"=w290:bool)
        n128 = call <vilib>:"Clear Errors.vi"("error in (no error)"=w293) -> ("error out"=w294:errorcluster)  [unwired: 5 in, 1 out]
        n129 = Select(t="FAILED", s=w290, f="SUCCESS") -> (s? t:f=w287:string)
        n130 = Format Into String(format string="Step '%s' completed with error code %d (%s)", w301, w291, w287) -> (resulting string=w300:string)  [unwired: 2 in, 1 out]
        n131 = Insert Into Array(array=w304, new element=w300) -> (w303:string[])  [unwired: 1 in]
        n132 = property on="BUILDER STATUS" class="LstBox (strict)"("Item Names"=w303) -> ()  [unwired: 2 in, 2 out]
        n133 = call <vilib>:"Add State(s) to Queue__jki_lib_state_machine.vi"("State(s) in (\"\")"=w310) -> ("States Out"=w309:string)  [unwired: 14 in]
      }
      frame "Build: Windows Volta Control Suite EXE" {
        w320 = "My Computer"  # Windows Build
        n134 = property on="BUILDER STATUS" class="LstBox (strict)"() -> ("Item Names"=w331:string[])  [unwired: 2 in, 2 out]
        n135 = Format Into String(format string="Running '%s' ...", w325) -> (resulting string=w329:string)  [unwired: 2 in, 1 out]
        n136 = Insert Into Array(array=w331, new element=w329) -> (w328:string[])  [unwired: 1 in]
        n137 = property on="BUILDER STATUS" class="LstBox (strict)"("Item Names"=w328) -> ()  [unwired: 2 in, 2 out]
        n138 = Current VI's Path() -> (path=w323:path)
        n139 = Strip Path(path=w323) -> (stripped path=w322:path)  [unwired: 1 out]
        n140 = Build Path(base path=w322, name or relative path="Volta Control Suite (Windows).lvproj") -> (appended path=w319:path)
        n141 = call-poly <vilib>:"Build.vi"("error in (no error)"=w316, "Name of target (My Computer)"=w320, "Path to project"=w319) -> ("error out"=w317:errorcluster)  [unwired: 7 in, 1 out]
        n142 = Unbundle By Name(w317) -> ("code"=w315:i32, "status"=w314:bool)
        n143 = call <vilib>:"Clear Errors.vi"("error in (no error)"=w317) -> ("error out"=w318:errorcluster)  [unwired: 5 in, 1 out]
        n144 = Select(t="FAILED", s=w314, f="SUCCESS") -> (s? t:f=w311:string)
        n145 = Format Into String(format string="Step '%s' completed with error code %d (%s)", w325, w315, w311) -> (resulting string=w324:string)  [unwired: 2 in, 1 out]
        n146 = Insert Into Array(array=w328, new element=w324) -> (w327:string[])  [unwired: 1 in]
        n147 = property on="BUILDER STATUS" class="LstBox (strict)"("Item Names"=w327) -> ()  [unwired: 2 in, 2 out]
        n148 = call <vilib>:"Add State(s) to Queue__jki_lib_state_machine.vi"("State(s) in (\"\")"=w334) -> ("States Out"=w333:string)  [unwired: 14 in]
      }
    }
  }
